vi "AB_API Set Destination Preserve Hierarchy.vi"(8 "error in (no error)":errorcluster, 9 "Preserve Hierarchy":bool, 10 "Destination label":string, 11 "Build in":refnum<class "AB_Build.lvclass">) -> (0 "error out":errorcluster, 3 "Build out":refnum<class "AB_Build.lvclass">)   [LabVIEW 2020]
uses:
  <vilib>/AppBuilder/AB_Classes/Build/AB_Build.lvclass
  <vilib>/AppBuilder/AB_Classes/Destination/AB_Destination.lvclass
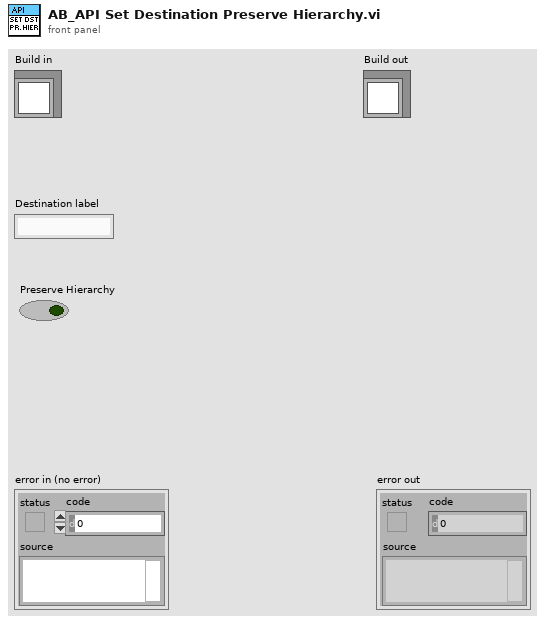
[diagram p1: front panel]
types:
  T1 = typedef "AB_Build.ctl" = cluster{"buildSpecName":string, "buildSpecDescription":string, "destinations":refnum<class "AB_Destination.lvclass">[], "exclusionOption":T2, "defaultLanguage":string, "supportedLanguages":string[], "excludedDirectories":path[], "buildContext":refnum<vi>, "buildObject":T3, "preview":bool, "programatic":bool, "progressBarEvents":T4, "userLog_Path":path, "preActionID":string, "preAction_Path":path, "postActionID":string, "postAction_Path":path, "eng_checkForBrokenVIs?":bool, "eng_verboseLinkerErrors?":bool, "localDest_Path":path, "targetDest_Path":path, "removeVIObject":u16, "cache":refnum<class "PreviewCache.lvclass">, "use cache":bool, "previewCache_ID":string, "buildCache_ID":string, "eng_TempLocalDest_Path":path, "eng_collectDependencies?":bool, "versionInfo":cluster{"buildVersion":cluster{"major":u16, "minor":u16, "patch":u16, "build":u16}, "autoIncrement":bool}, "eng_enableVIChecksums":bool}
  T2 = typedef "AB_Exclusion_Option.ctl" = cluster{"typedefs":bool, "polymorphicVIs":bool, "unusedLibraryItems":bool, "modifyLibraryFile":bool, "edit-timeDependencies":bool, "inlineVIs":bool, "dependent PPLs":bool, "dependent DLLs":bool}
  T3 = typedef "ItemRef.ctl" = u64
  T4 = typedef "provcom_ProgressBar_Events.ctl" = cluster{"newJob":refnum<user-event>, "newItem":refnum<user-event>, "errorMsg":T5, "cancel":refnum<user-event>}
  T5 = typedef "mxLvBuildError.ctl" = refnum<user-event>
  T6 = typedef "AB_Destination.ctl" = cluster{"destName":string, "path":path, "libraryName":string, "preserveHierarchy":bool, "eng_inBuild":bool, "eng_libraryReference":refnum<vi>, "eng_restictAddToNewLibrary":bool}
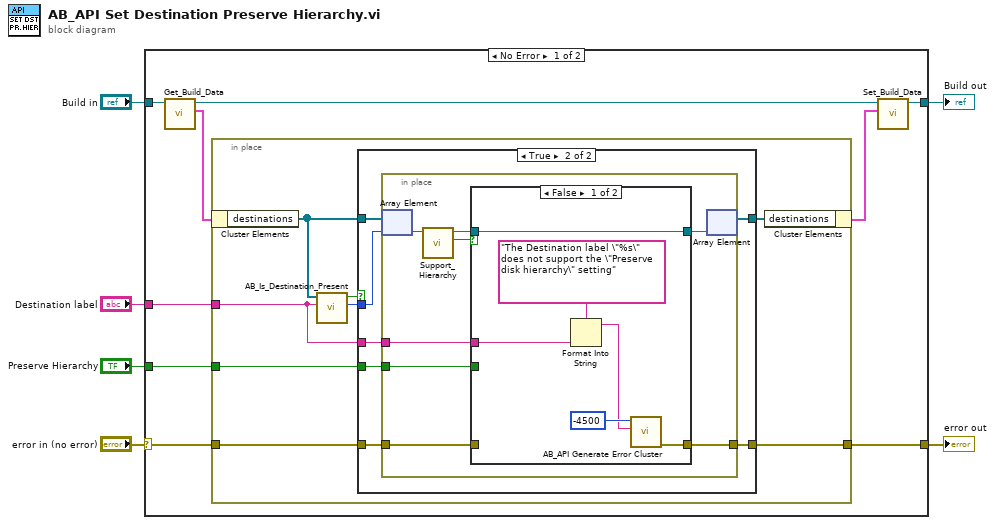
[diagram p0: block diagram]
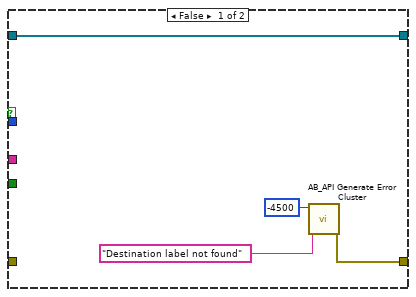
[diagram p2: hidden frame]
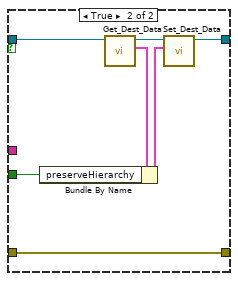
[diagram p3: hidden frame]
diagram:
  n1 = case shown="No Error" "error in (no error)" {
    selector: "error in (no error)" -> [w14 w57]
    tunnel: [w13 w57] -> w5
    tunnel: "Destination label" -> [w15 _]
    tunnel: "Preserve Hierarchy" -> [w11 _]
    tunnel: [w7 w56] -> w2
    tunnel: "Build in" -> [w12 w56]
    frame No Error {
      n2 = call <vilib>:"Get_Build_Data.vi"("Class in"=w12) -> ("data"=w9:T1, "Class out"=w10:refnum<class "AB_Build.lvclass">)  [unwired: 1 in, 8 out]
      n3 = in-place {
        in-place-border: w15 -> [w16]
        in-place-border: w11 -> [w22]
        in-place-border: [w20] -> w13
        in-place-border: w14 -> [w19]
        n4 = in-place-cluster #1(w9) -> ("destinations"=w17:refnum<class "AB_Destination.lvclass">[])
        n5 = call <vilib>:"AB_Is_Destination_Present.vi"("destination label"=w16, "destinations"=w17) -> ("index"=w18:i32, "destination present?"=w21:bool)  [unwired: 3 in, 5 out]
        n6 = case shown="True" w21 {
          tunnel: w17 -> [w27 w34]
          tunnel: [w27 w33] -> w23
          tunnel: w18 -> [_ w32]
          tunnel: w22 -> [_ w31]
          tunnel: [w24 w29] -> w20
          tunnel: w19 -> [_ w30]
          tunnel: w16 -> [_ w28]
          frame False {
            n7 = call <vilib>:"AB_API Generate Error Cluster.vi"("Additional Message"="Destination label not found", "Code"=-4500) -> ("error out"=w24:errorcluster)  [unwired: 2 in, 7 out]
          }
          frame True {
            n8 = in-place {
              in-place-border: w31 -> [w42]
              in-place-border: w30 -> [w38]
              in-place-border: [w36] -> w29
              in-place-border: w28 -> [w35]
              n9 = in-place-array #2(w34, w32) -> (w40:refnum<class "AB_Destination.lvclass">)
              n10 = call-dynamic "Support_Hierarchy.vi"("AB_Destination in"=w40) -> ("support hierarchy"=w37:bool, "AB_Destination out"=w39:refnum<class "AB_Destination.lvclass">)  [unwired: 8 in, 1 out]
              n11 = case shown="False" w37 {
                tunnel: w42 -> [_ w54]
                tunnel: [w48 w52] -> w41
                tunnel: w39 -> [w48 w50]
                tunnel: w38 -> [_ w49]
                tunnel: [w46 w49] -> w36
                tunnel: w35 -> [w43 _]
                frame False {
                  n12 = Format Into String(format string="The Destination label \"%s\" does not support the \"Preserve disk hierarchy\" setting" ("Additional Message"), w43) -> (resulting string=w44:string)  [unwired: 2 in, 1 out]
                  n13 = call <vilib>:"AB_API Generate Error Cluster.vi"("Additional Message"=w44, "Code"=-4500) -> ("error out"=w46:errorcluster)  [unwired: 2 in, 7 out]
                }
                frame True {
                  n14 = call <vilib>:"Get_Dest_Data.vi"("Class in"=w50) -> ("destName"=w55:T6, "Class out"=w53:refnum<class "AB_Destination.lvclass">)  [unwired: 1 in, 8 out]
                  n15 = Bundle By Name(cluster=w55, "preserveHierarchy"=w54) -> (w51:T6)
                  n16 = call <vilib>:"Set_Dest_Data.vi"("destName"=w51, "Class in"=w53) -> ("Class out"=w52:refnum<class "AB_Destination.lvclass">)  [unwired: 8 in, 1 out]
                }
              }
              n17 = in-place-array #2(w41) -> (w33:refnum<class "AB_Destination.lvclass">[])  [unwired: 1 out]
            }
          }
        }
        n18 = in-place-cluster #1("destinations"=w23) -> (w8:T1)
      }
      n19 = call <vilib>:"Set_Build_Data.vi"("data"=w8, "Class in"=w10) -> ("Class out"=w7:refnum<class "AB_Build.lvclass">)  [unwired: 1 in, 8 out]
    }
    frame Error {
    }
  }
  "error out" <- w5
  "Build out" <- w2
